vi "getLastPublishedTimeoutActuatorIds.vi"(11 "Publisher in":refnum<class "Publisher.lvclass">) -> (2 "LastPublishedTimeoutActuatorIds":i32[](array[numeric]), 3 "Publisher out":refnum<class "Publisher.lvclass">)   [LabVIEW 2016, in "Publisher.lvclass"]
uses:
  Publisher.lvclass
  Publisher.lvclass/Publisher.ctl
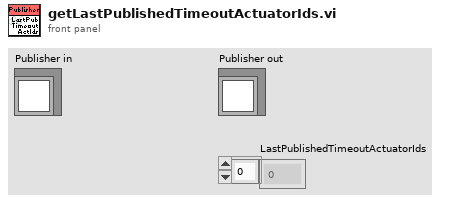
[diagram p1: front panel]
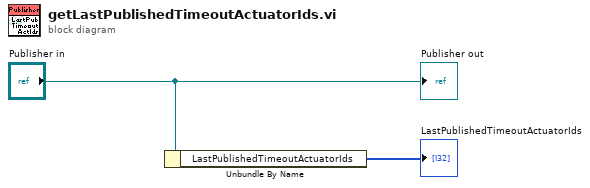
[diagram p0: block diagram]
diagram:
  n1 = Unbundle By Name("Publisher in") -> ("LastPublishedTimeoutActuatorIds"=→"LastPublishedTimeoutActuatorIds":i32[])
  "Publisher out" <- "Publisher in"
